vi "set_shutter.vi"(11 "open?":bool) -> ()   [LabVIEW 2011]
uses:
  <vilib>/rvi/eio/common/nirviEmuTemplateMethod_errors.vi
  <vilib>/eio/EIONode/EIONode.xnode
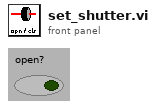
[diagram p1: front panel]
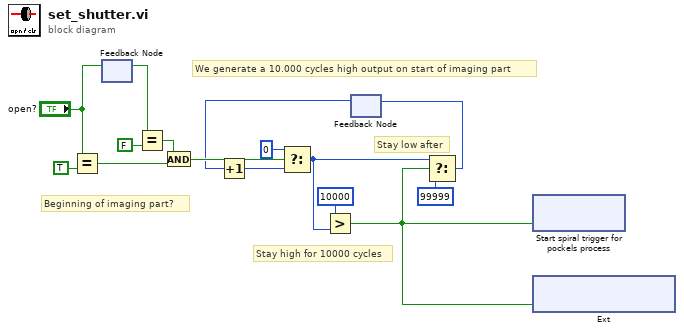
[diagram p0: block diagram]
diagram:
  # "Stay low after"
  # "Stay high for 10000 cycles"
  # "Beginning of imaging part?"
  # "We generate a 10.000 cycles high output on start of imaging part"
  n1 = Equal?(x="open?", y=TRUE) -> (x = y?=w10:bool)
  n2 = feedback #1() -> (w13:bool)  [unwired: 1 in]
  n3 = feedback-in #1("open?") -> ()
  n4 = Equal?(x=w13, y=FALSE) -> (x = y?=w11:bool)
  n5 = And(x=w11, y=w10) -> (x .and. y?=w7:bool)
  n6 = feedback #2() -> (w3:u32)  [unwired: 1 in]
  n7 = Increment(x=w3) -> (x+1=w8:u32)
  n8 = Select(t=u32 0, s=w7, f=w8) -> (s? t:f=w5:u32)
  n9 = Greater?(x=u32 10000, y=w5) -> (0:w1:bool)
  n10 = Select(t=w5, s=w1, f=u32 99999) -> (s? t:f=w4:u32)
  n11 = feedback-in #2(w4) -> ()
  n12 = xnode "Start spiral trigger for pockels process"("PXI_Trig0"=w1) -> ()  [unwired: 1 in, 1 out]
  n13 = xnode "Ext"("Connector0/DIO32"=w1) -> ()  [unwired: 1 in, 1 out]
